vi "Robot Global Data.vi"() -> ()   [LabVIEW 2014]
doc: "This global VI can contain as many global variables as you need. Place a control on the panel, give it a good name. To read or write to it from a VI, drag the icon to the diagram of that VI. You can also drag from the project. Click on the node to change which global you access. You shouldn't have multiple locations writing to a global or it will cause a race-condition."
uses:
  <vilib>/Rock Robotics/WPI/DriverStation/WPI_DriverStationRobotMode2.ctl
panel:
  in  "Disable Coordinate Setting":bool
  out "Wrist Invert":bool
  out "Extension Invert":bool
  out "Pivot Invert":bool
  out "Wheel Angle Invert":bool
  in  "Y Target":dbl
  in  "X Target":dbl
  in  "Pivot Target":dbl
  in  "Extension Target":dbl
  in  "Wrist Motor Height":dbl=5.5
  in  "Claw Angle with Bin":dbl
  in  "Holding Bin":bool
  in  "Claw State":enum16{"Open", "Closed", "Neither"}(ring)
  in  "Extension Soft Limits":cluster{"Forward":dbl, "Reverse":dbl}
  in  "Claw Soft Limits":cluster{"Forward":dbl, "Reverse":dbl}
  in  "Wrist Soft Limits":cluster{"Forward":dbl, "Reverse":dbl}
  in  "Pivot Soft Limits":cluster{"Forward":dbl, "Reverse":dbl}
  in  "Claw Offset":dbl
  in  "Camera Offset (x)":dbl=-7.0
  in  "Camera Offset (y)":dbl=2.75
  in  "y Coordinate of Bin":dbl=2.25
  in  "x Coordinate of Bin":dbl=5.25
  in  "Max Extention Without Tipping With Bin":dbl
  in  "Vision Ratio":dbl
  in  "Vision Distance":dbl
  in  "Vision Angle":dbl
  in  "Drive Train Absolute Offsets (ticks)":dbl[](array[numeric])=[-0.395, 1.11, 1.68, -1.896]
  in  "Drive Train Wheel Angles (rad)":cluster{"FL":dbl, "FR":dbl, "RL":dbl, "RR":dbl}={"FL"=-0.395, "FR"=1.11, "RL"=1.68, "RR"=-1.896}
  in  "Coordinates":cluster{"X":dbl, "Y":dbl, "Heading":dbl}={"X"=0.0, "Y"=0.0, "Heading"=90.0}
  in  "Wheel Speed TPI":dbl=2292.3908 format="%#_10g"
  in  "Rumble":cluster{"Intensity":dbl, "Duration":i16}={"Intensity"=0.0, "Duration"=10}
  in  "Claw Open / Close (F / T)":bool
  in  "Pivot Offset":dbl
  in  "Wrist Offset":dbl
  in  "Segment One Length":dbl=37.5
  in  "Wrist Target":dbl
  in  "Extend TPI":dbl=98.0392156863 format="%#_20g"
  in  "Absolute Encoder TPR":dbl=162.97466
  in  "Claw Length":dbl=25.0
  in  "Max Height":dbl=54.0
  in  "Robot Width":dbl=24.5
  in  "Robot Length":dbl=24.5
  in  "Robot Mode":T1
  # "Ticks Per Radian"
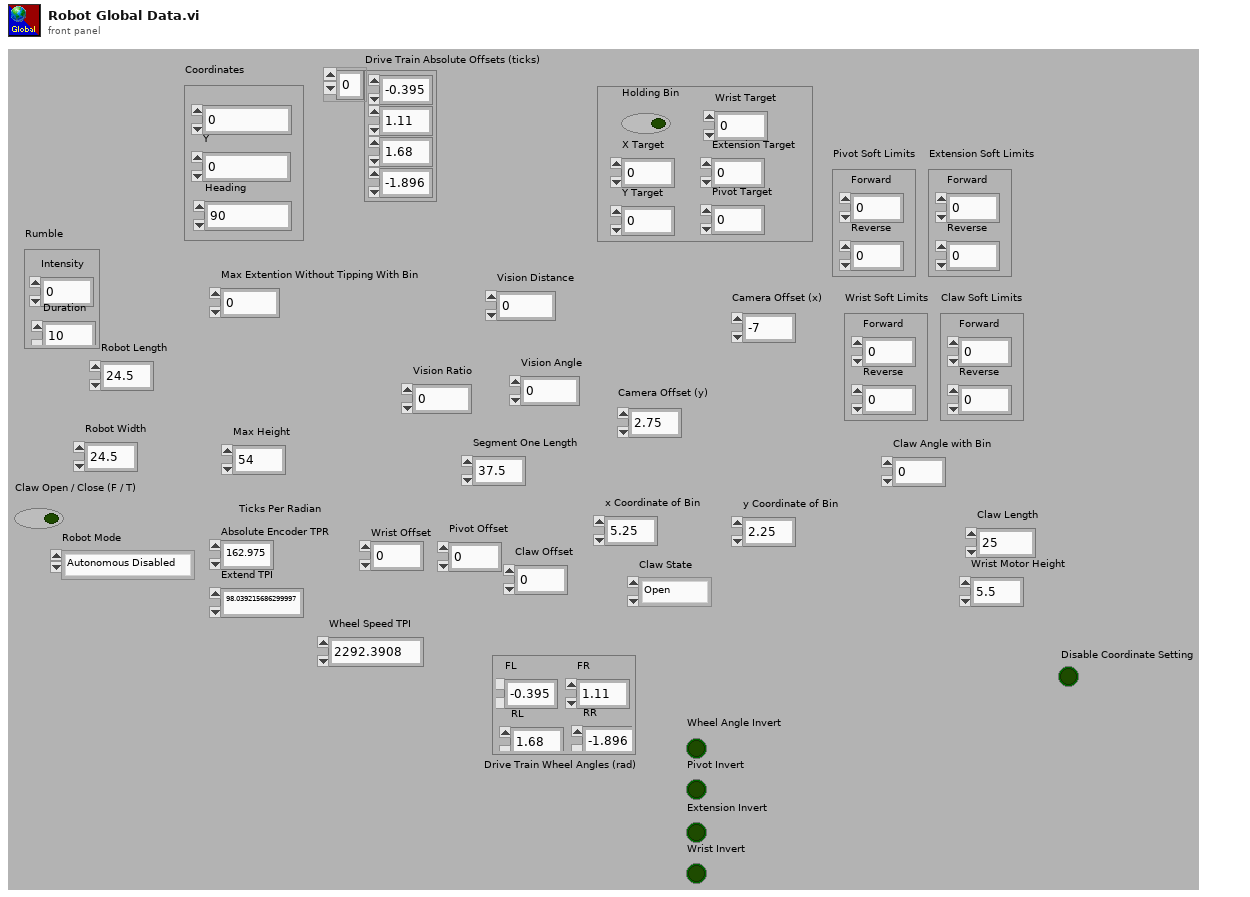
[diagram p1: front panel]
types:
  T1 = typedef "WPI_DriverStationRobotMode2.ctl" = enum16{"Autonomous Disabled", "Autonomous Enabled", "Teleop Disabled", "Teleop Enabled", "Disconnected", "Finish", "Test Disabled", "Test Enabled", "Emergency Stopped"}
diagram:
